vi "Commit NIRFSG.vi"(8 "error in":errorcluster, 11 "PAE Reference In":T1) -> (0 "error out":errorcluster, 3 "PAE Reference Out":T1)   [LabVIEW 2023]
uses:
  <vilib>/niPAEML/Typedefs/Session Handle.ctl
  <vilib>/niPAEML/PAE Reference.lvclass
  <vilib>/niPAEML/PAE Reference.lvclass/PAE Reference.ctl
  <vilib>/niPAEML/PAE/Datatypes/Pulse Trigger to Export.ctl
  <vilib>/niPAEML/Accessors/Read RFSG Pulse Trigger Output Terminal.vi
  <vilib>/niPAEML/Accessors/Read RFSG to RFmx Trigger Routing Mode.vi
  <vilib>/niPAEML/Accessors/Read RFSG Trigger Output Type.vi
  <vilib>/niPAEML/Accessors/Read NI DCPower Channel Name.vi
  <vilib>/niPAEML/Accessors/Read NI DCPower Instrument Handle.vi
  <vilib>/niPAEML/Accessors/Read RFSG Pulse Trigger Input Terminal.vi
  <vilib>/niPAEML/Accessors/Read DCPower Stimulus Mode.vi
  <vilib>/niPAEML/Accessors/Read RFSG Pulse Trigger Delay (s).vi
  <vilib>/niPAEML/Accessors/Read RFSG PRI (s).vi
  <vilib>/niPAEML/Accessors/Read RFSG Pulse Width (s).vi
  <vilib>/niPAEML/Accessors/Read RFSG Post-trigger Time (s).vi
  <vilib>/niPAEML/Accessors/Read RFSG Pre-trigger Time (s).vi
  <vilib>/niPAEML/Accessors/Read NI RFSG Session.vi
  <vilib>/niPAEML/Accessors/Read NI RFSG Port.vi
  <vilib>/niPAEML/Accessors/Read RFSG Stimulus Mode.vi
  <vilib>/niPAEML/Accessors/Read Initial Power (dBm).vi
  <vilib>/niPAEML/Accessors/Read Tx Start Frequency (Hz).vi
  <vilib>/niPAEML/Utilities/Shared/PAE Shared.lvlib
  <vilib>/niPAEML/PAE/PAEML.lvlib
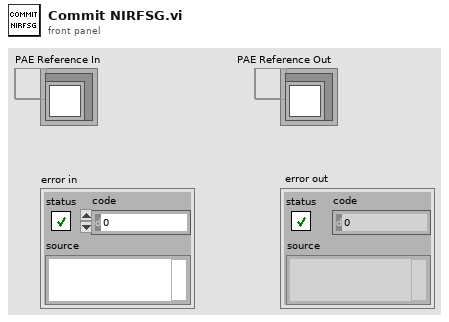
[diagram p1: front panel]
types:
  T1 = typedef "PAE Measurement.lvlib/PAE Reference.lvclass/Session Handle.ctl" = refnum<data-value>
  T2 = typedef "PAEML.lvlib/Pulse Trigger to Export.ctl" = enum16{"None", "Pulse", "Gate", "Gate+Pulse"}
  T3 = typedef "PAE Measurement.lvlib/PAE Reference.lvclass/RFSG Stimulus Mode.ctl" = enum16{"CW", "Pulsed CW"}
  T4 = typedef "niRFSG Exported Signal Destinations.ctl" = string
  T5 = typedef "PAE Measurement.lvlib/PAE Reference.lvclass/Trigger Routing Mode.ctl" = enum16{"Automatic", "Manual"}
  T6 = typedef "PAE Measurement.lvlib/PAE Reference.lvclass/Trigger Type.ctl" = enum16{"Pulse", "Gate"}
  T7 = typedef "PAE Measurement.lvlib/PAE Reference.lvclass/RFSG Trigger Input Terminal.ctl" = string
  T8 = typedef "PAE Measurement.lvlib/PAE Reference.lvclass/DCPower Stimulus Mode.ctl" = enum16{"Constant", "Pulsed"}
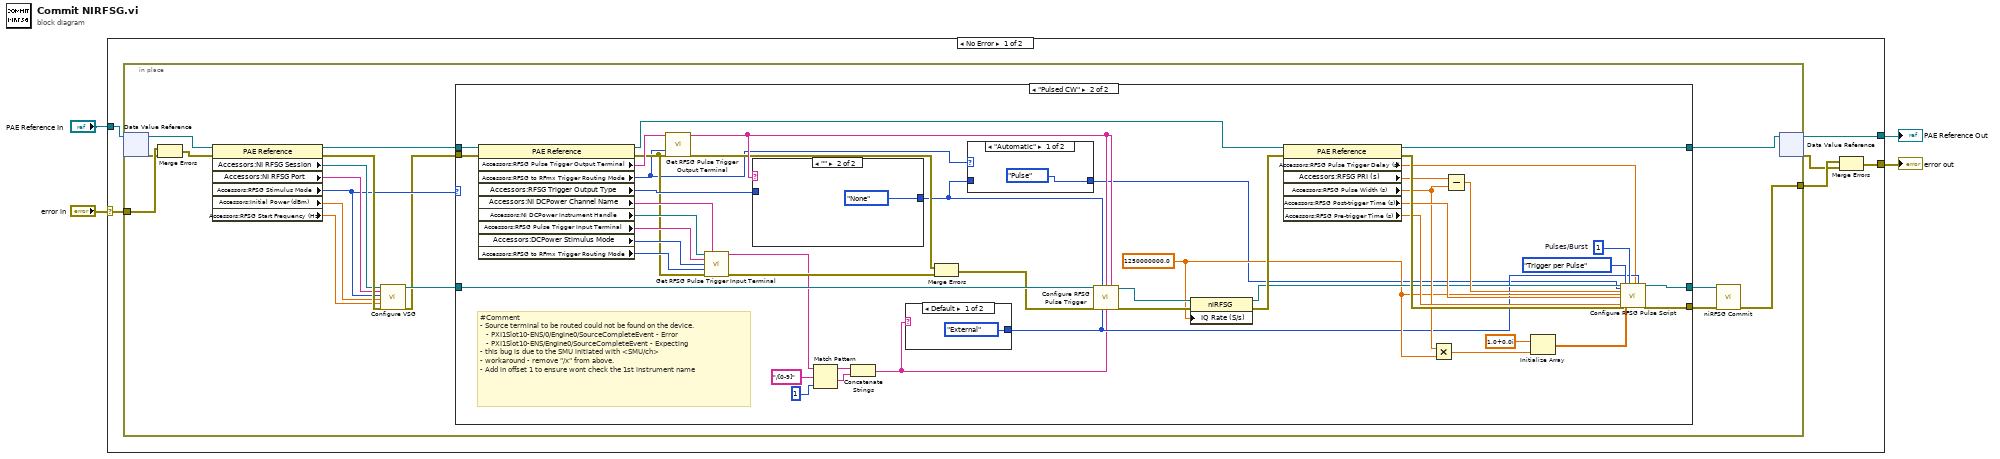
[diagram p0: block diagram]
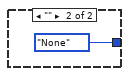
[diagram p4: hidden frame]
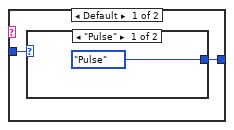
[diagram p5: hidden frame]
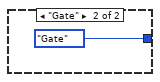
[diagram p6: hidden frame]
diagram:
  n1 = case shown="No Error" "error in" {
    selector: "error in" -> [w10 w87]
    tunnel: "PAE Reference In" -> [w6 w86]
    tunnel: [w5 w86] -> w1
    tunnel: [w7 w87] -> w4
    frame No Error {
      n2 = in-place {
        in-place-border: w10 -> [w27]
        in-place-border: [w14] -> w9
        n3 = in-place-dvr #1(w6) -> (w21:refnum<class "PAE Reference.lvclass">, w26:errorcluster)
        n4 = Merge Errors(w27, w26) -> (w11:errorcluster)
        n5 = property class="PAE Reference"(reference=w21, error in=w11) -> (reference out=w18:refnum<class "PAE Reference.lvclass">, error out=w25:errorcluster, "Accessors:NI RFSG Session"=w20:refnum<k15>, "Accessors:NI RFSG Port"=w24:string, "Accessors:RFSG Stimulus Mode"=w13:T3, "Accessors:Initial Power (dBm)"=w23:dbl, "Accessors:RFSG Start Frequency (Hz)"=w22:dbl)
        n6 = call "Configure VSG.vi"("instrument handle in"=w20, "RFSG port"=w24, "RFSG Stimulus Mode"=w13, "power level (dBm)"=w23, "frequency (Hz)"=w22, "error in"=w25) -> ("instrument handle out"=w19:refnum<k15>, "error out"=w12:errorcluster)  [unwired: 12 in]
        n7 = case shown="\"Pulsed CW\"" w13 {
          tunnel: w12 -> [w29 w76]
          tunnel: w19 -> [w28 w75]
          tunnel: w18 -> [w30 w74]
          tunnel: [w30 w59] -> w17
          tunnel: [w29 w58] -> w16
          tunnel: [w28 w57] -> w15
          frame "CW" {
          }
          frame "Pulsed CW" {
            w52 = 1250000000.0
            w68 = 1  # Pulses/Burst
            # "#Comment\n- Source terminal to be routed could not be found on the device.\n   - PXI1Slot10-ENS/0/Engine0/SourceCompleteEvent - Error\n   - PXI1Slot10-ENS/Engine0/SourceCompleteEvent - Expecting\n- this bug is due to the SMU initiated with <SMU/ch> \n- workaround - remove \"/x\" from above.\n- Add in offset 1 to ensure wont check the 1st instrument name"
            n8 = property class="PAE Reference"(reference=w74, error in=w76) -> (reference out=w70:refnum<class "PAE Reference.lvclass">, error out=w46:errorcluster, "Accessors:RFSG Pulse Trigger Output Terminal"=w73:T4, "Accessors:RFSG to RFmx Trigger Routing Mode"=w39:T5, "Accessors:RFSG Trigger Output Type"=w72:T6, "Accessors:NI DCPower Channel Name"=w51:string, "Accessors:NI DCPower Instrument Handle"=w50:refnum<k15>, "Accessors:RFSG Pulse Trigger Input Terminal"=w49:T7, "Accessors:DCPower Stimulus Mode"=w48:T8, "Accessors:RFSG to RFmx Trigger Routing Mode"=w47:T5)
            n9 = call <vilib>:"Get RFSG Pulse Trigger Output Terminal.vi"("User Specified RFSG Pulse Trigger Output Terminal"=w73, "RFSG to RFmx Trigger Routing Mode"=w39, "error in"=w46) -> ("RFSG Pulse Trigger Output Terminal"=w71:T4, "error out"=w45:errorcluster)  [unwired: 11 in]
            n10 = call <vilib>:"Get RFSG Pulse Trigger Input Terminal.vi"("DCPower Instrument Handle"=w50, "DCPower Channel"=w51, "User Specified RFSG Pulse Trigger Input Terminal"=w49, "DCPower Stimulus Mode"=w48, "DCPower to RFSG Trigger Routing Mode"=w47, "error in"=w46) -> ("RFSG Pulse Trigger Input Terminal"=w35:T7, "error out"=w44:errorcluster)  [unwired: 8 in]
            n11 = case shown="\"\"" w71 {
              tunnel: w72 -> [w82 _]
              tunnel: [w81 Pulse_Trigger_to_Export."None" ("triggers to export")] -> w38
              frame Default {
                n12 = case shown="\"Pulse\"" w82 {
                  tunnel: [Pulse_Trigger_to_Export."Pulse" ("triggers to export") Pulse_Trigger_to_Export."Gate" ("triggers to export")] -> w81
                  frame "Pulse" {
                  }
                  frame "Gate" {
                  }
                }
              }
              frame "" {
              }
            }
            n13 = Match Pattern(string=w35, regular expression="/[0-9]", offset (0)=1) -> (before substring=w34:T7, after substring=w33:T7)  [unwired: 2 out]
            n14 = Concatenate Strings(w34, w33) -> (w32:string)
            n15 = case shown="Default" w32 {
              tunnel: [enum32{"None", "External"}."External" ("import trigger parameters") enum32{"None", "External"}."None" ("import trigger parameters")] -> w43
              frame Default {
              }
              frame "" {
              }
            }
            n16 = Merge Errors(w45, w44) -> (w40:errorcluster)
            n17 = case shown="\"Automatic\"" w39 {
              tunnel: w38 -> [_ w78]
              tunnel: [Pulse_Trigger_to_Export."Pulse" ("triggers to export") w78] -> w37
              frame "Automatic" {
              }
              frame "Manual" {
              }
            }
            n18 = call <vilib>:"Configure RFSG Pulse Trigger.vi"("IVI Refnum in"=w75, "triggers to export"=w38, "gate trigger destination"=w71, "pulse/env trigger destination"=w71, "error in"=w40, "import trigger parameters"=w43, "external trigger source"=w32) -> ("IVI Refnum out"=w55:refnum<k15>, "error out"=w56:errorcluster)  [unwired: 6 in, 1 out]
            n19 = property class="niRFSG"(reference=w55, error in=w56, "IQ Rate (S/s)"=w52) -> (reference out=w53:refnum<k15>, error out=w54:errorcluster)
            n20 = property class="PAE Reference"(reference=w70, error in=w54) -> (reference out=w59:refnum<class "PAE Reference.lvclass">, error out=w69:errorcluster, "Accessors:RFSG Pulse Trigger Delay (s)"=w41:dbl, "Accessors:RFSG PRI (s)"=w42:dbl, "Accessors:RFSG Pulse Width (s)"=w63:dbl, "Accessors:RFSG Post-trigger Time (s)"=w65:dbl, "Accessors:RFSG Pre-trigger Time (s)"=w64:dbl)
            n21 = Multiply(x=w63, y=w52) -> (x*y=w62:dbl)
            n22 = Subtract(x=w42, y=w63) -> (x-y=w66:dbl)
            n23 = Initialize Array(cdb 1.0+0.0i, w62) -> (w60:cdb[])
            n24 = call <vilib>:"Configure RFSG Pulse Script.vi"("IVI Refnum in"=w53, "Triggers to Export"=w37, "Blank duration (s)"=w66, "Generation IQ rate (S/s)"=w52, "Export Post-trig Time (s)"=w65, "Export Pretrigger Time (s)"=w64, "error in"=w69, "Trig Type"=enum16{"Trigger per Pulse", "Trigger per Burst"}."Trigger per Pulse", "Wave Input"=w60, "#Pulses/Burst"=w68, "Trigger Delay (s)"=w41, "Import Trigger Parameters"=w43) -> ("IVI Refnum out"=w57:refnum<k15>, "error out"=w58:errorcluster)  [unwired: 13 in, 1 out]
          }
        }
        n25 = call <instrlib>:"niRFSG Commit.vi"("instrument handle"=w15, "error in"=w16) -> ("error out"=w14:errorcluster)  [unwired: 12 in, 1 out]
        n26 = in-place-dvr #1(w17) -> (w5:T1, w8:errorcluster)
      }
      n27 = Merge Errors(w9, w8) -> (w7:errorcluster)
    }
    frame Error {
    }
  }
  "PAE Reference Out" <- w1
  "error out" <- w4
